vi "Send RemoveShap Event (Poly).vi"   [LabVIEW 2017, in "LV Image Editor Framework.lvlib" / "Image Editor Handler.lvclass"]
uses:
  <vilib>/LIEF/Image Editor Handler/Image Editor Handler.lvclass
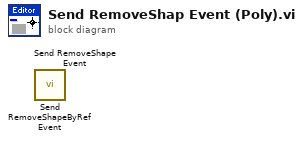
[diagram p0: block diagram]
diagram:
  n1 = call <vilib>:"Send RemoveShapeByRef Event.vi"() -> ()  [unwired: 10 in, 2 out]
  n2 = call <vilib>:"Send RemoveShape Event.vi"() -> ()  [unwired: 10 in, 2 out]
